vi "Globali.vi"() -> ()   [LabVIEW 2022 SP3]
panel:
  out "Fase Prot35":bool
  out "Fase Scarico":bool
  out "I.A. 4":bool
  out "I.A. 3":bool
  out "I.A. 2":bool
  out "I.A. 1":bool
  in  "copia dati report":string[](array[string])
  in  "Dati_report":string[](array[string])
  in  "Ore manut.":i16
  in  "Militare":bool
  out "t. tot.":i32 format="%<%H:%M:%S>t"
  out "t. Step":i32 format="%<%H:%M:%S>t"
  out "PASS MAN.":string
  in  "Tipo":i16
  out "F.1_NOK_PERDITE_OLIO":bool
  out "F.1_OK_PERDITE_OLIO":bool
  out "PR.1_OK_RUMORE":bool
  out "prod/ric/rev":string
  out "PASS OPER.":string
  out "PASS AMM.":string
  out "m_tipo":u32
  out "m_start":bool
  out "m_tempo":bool
  out "m_numero cicli":bool
  out "m_1 avvio":bool
  out "Scrivi":bool
  in  "Autocontrollo":string
  out "In?":bool
  out "Indicazioni":string
  out "O.F.2-2_OK_LAVAGGIO":bool
  out "O.F.2-1_OK_EROGAZ_PROT35":bool
  out "O.F.3_OK_FINE_CICLO":bool
  out "O.F.1-1_OK_EROGAZ_PROD":bool
  out "I.A.2_OK_FLANGIA_BLOCC":bool
  out "I.A.1_OK_FLANGIA_LIBERA":bool
  out "O.P.3_OK_INSER_ASSE":bool
  out "O.P.2_OK_RISCALDO":bool
  out "O.P.1_OK_EROGAZIONE":bool
  out "Directory modelli report":path=path "D:/Archivio/Iveco/074-07/LabView/Appoggio"
  in  "diagnostica":bool
  out "Testo allarmi":string caption="Collaudo in corso"
  out "Testo fase collaudo":string caption="Collaudo in corso"
  out "Testo segnalazioni":string caption="Collaudo in corso"
  out "Testo messaggi":string caption="Collaudo in corso"
  in  "Tab Control":enum32{"SCRITTURA", "LETTURA"}(tab)=enum."LETTURA"
  in  "226. 0":sgl min=0 format="%.2f"
  in  "230. 0":sgl min=0 format="%.2f"
  in  "Calibrazione torsiometro":sgl min=0 format="%.2f"
  in  "VERNICIATO":bool
  in  "OK_MANUTENZIONE":bool
  in  "CONTINUA PROVA":bool
  in  "SOSPENDI PROVA":bool
  in  "ANNULLA PROVA":bool
  in  "2. 5":bool
  in  "0. 0":bool
  in  "0. 1":bool
  in  "0. 2":bool
  in  "0. 3":bool
  in  "0. 4":bool
  in  "0. 5":bool
  in  "0. 6":bool
  in  "0. 7":bool
  in  "1. 0":bool
  in  "1. 1":bool
  in  "1. 2":bool
  in  "1. 3":bool
  in  "1. 4":bool
  in  "1. 5":bool
  in  "1. 6":bool
  in  "1. 7":bool
  in  "2. 0":bool
  in  "2. 1":bool
  in  "2. 2":bool
  in  "2. 3":bool
  in  "2. 4":bool
  in  "4. 0":i16(ring) items=["PRODOTTO", "RP3000", "AAT 2", "AAT 1 3 4"]
  in  "6. 0":i16(ring) items=["TIPO", "PRODUZIONE", "RICAMBIO"]
  in  "8. 0":i16 min=0
  in  "12. 0":sgl min=0 format="%.2f"
  in  "16. 0":i16 min=0
  in  "22. 0":sgl min=0 format="%.2f"
  in  "26. 0":sgl min=0 format="%.2f"
  in  "32. 0":sgl min=0 format="%.2f"
  in  "36. 0":sgl min=0 format="%.2f"
  in  "44. 0":i16 min=0
  in  "50. 0":i16 min=0
  in  "56. 0":i16 min=0
  in  "62. 0":i16 min=0
  in  "68. 0":i16 min=0
  in  "72. 0":sgl min=0 format="%.2f"
  in  "76. 0":sgl min=0 format="%.2f"
  in  "80. 0":sgl min=0 format="%.2f"
  in  "84. 0":i16 min=0
  in  "88. 0":sgl min=0 format="%.2f"
  in  "92. 0":sgl min=0 format="%.2f"
  in  "96. 0":sgl min=0 format="%.2f"
  in  "100. 0":i16 min=0
  in  "104. 0":sgl min=0 format="%.2f"
  in  "108. 0":sgl min=0 format="%.2f"
  in  "112. 0":sgl min=0 format="%.2f"
  in  "116. 0":i16 min=0
  in  "120. 0":sgl min=0 format="%.2f"
  in  "124. 0":sgl min=0 format="%.2f"
  in  "128. 0":sgl min=0 format="%.2f"
  in  "134. 0":sgl min=0 format="%.2f"
  in  "138. 0":sgl min=0 format="%.2f"
  in  "144. 0":i16 min=0
  in  "148. 0":i16 min=0
  in  "154. 0":i16 min=0
  in  "160. 0":sgl min=0 format="%.2f"
  in  "164. 0":sgl min=0 format="%.2f"
  in  "168. 0":sgl min=0 format="%.2f"
  in  "172. 0":i16 min=0
  in  "176. 0":sgl min=0 format="%.2f"
  in  "180. 0":sgl min=0 format="%.2f"
  in  "184. 0":sgl min=0 format="%.2f"
  in  "190. 0":sgl min=0 format="%.2f"
  in  "194. 0":sgl min=0 format="%.2f"
  in  "200. 0":i16 min=0
  in  "206. 0":i16 min=0
  in  "212. 0":i16 min=0
  in  "20. 0":u16
  in  "30. 0":u16
  in  "40. 0":u16
  in  "42. 0":u16
  in  "48. 0":u16
  in  "54. 0":u16
  in  "60. 0":u16
  in  "66. 0":u16
  in  "132. 0":u16
  in  "142. 0":u16
  in  "152. 0":u16
  in  "158. 0":u16
  in  "188. 0":u16
  in  "198. 0":u16
  in  "204. 0":u16
  in  "210. 0":u16
  in  "216. 0":u16
  in  "218. 0":u16
  out "S_VERNICIATO":bool
  out "CICLO_IN_CORSO":bool
  out "S_SCARTO":bool
  out "Cicli_macchina":u16
  out "V_SOVRAPRESSIONE_DX":sgl format="%.2f"
  out "V_SOVRAPRESSIONE_SX":sgl format="%.2f"
  out "S_CANCELLI_CHIUSI":bool
  out "S_CANCELLI_APERTI":bool
  out "S_CARRO_IN_POSIZ_RP3000":bool
  out "S_FILTRO_INTASATO_PROT35":bool
  out "S_FILTRO_INTASATO_RICIRC":bool
  out "V_PERDITA_PRESSURIZZ_DX":sgl format="%.2f"
  out "V_PERDITA_PRESSURIZZ_SX":sgl format="%.2f"
  out "V_PERDITA_GONFIAGGIO_DX":sgl format="%.2f"
  out "V_PERDITA_GONFIAGGIO_SX":sgl format="%.2f"
  out "V_GONFIAGGIO_STAB":sgl format="%.2f"
  out "I1.0-2 EMERGENZA":bool
  out "S_CANCELLO_DX_APERTO":bool
  out "S_CANCELLO_SX_CHIUSO":bool
  out "S_CANCELLO_DX_CHIUSO":bool
  out "S_AUX_ON":bool=TRUE
  out "S_PRESSOSTATO_ARIA":bool
  out "S_CANCELLO_SX_APERTO":bool
  out "S_CANCELLO_SX_SBLOCCATO":bool
  out "S_CANCELLO_DX_SBLOCCATO":bool
  out "S_TRAZIONE_INSERITA":bool
  out "S_SCARICO_A_LAV":bool
  out "S_SCARICO_A_RIP":bool
  out "S_CARRELLO_10W30":bool
  out "S_CARRELLO_W90":bool
  out "S_CARRELLO_PROT35":bool
  out "S_SCARICO_B_LAV":bool
  out "S_SCARICO_B_RIP":bool
  out "S_CARRO_IN_POSIZ_AAT":bool
  out "S_MOTORE_FERMO":bool
  out "C_APERTURA_CANCELLI":bool
  out "C_START_PROVA":bool
  out "C_RESET":bool
  out "C_CHIUSURA_CANCELLI":bool
  out "C_FASE_SUCCESSIVA":bool
  out "S_ALLARME_INVERTER":bool
  out "S_LIVELLO_MIN_10W30":bool
  out "S_LIVELLO_MIN_W90":bool
  out "S_LIVELLO_MIN_PROT35":bool
  out "S_FILTRO_INTASATO_10W30":bool
  out "S_FILTRO_INTASATO_W90":bool
  out "S_PERDITA_10W30":bool
  out "S_PERDITA_W90":bool
  out "S_PERDITA_PROT35":bool
  out "S_TERMICA_10W30":bool
  out "S_TERMICA_W90":bool
  out "S_TERMICA_PROT35":bool
  out "S_TERMICA_RICIRCOLO":bool
  out "CARICO_ARIA_6_BAR":bool
  out "SCARICO_ARIA_6_BAR":bool
  out "CARICO_PRESSURIZZ":bool
  out "S_PERDITA_VASCA_RACCOLT":bool
  out "SCARICO_PRESSURIZZ":bool
  out "RICIRCOLO_OLIO":bool
  out "ACCENSIONE_AZIONAMENTO":bool
  out "START_MOTORE":bool
  out "POMPA_RICIRCOLO":bool
  out "SCARICO_B":bool
  out "EROGAZIONE_10W30":bool
  out "EROGAZIONE_W90":bool
  out "CHIUSURA_CANCELLI":bool
  out "APERTURA_CANCELLI":bool
  out "SCARICO_A":bool
  out "EROGAZIONE_PROT35":bool
  out "ROTAZIONE_SX":bool
  out "SBLOCCO_CANCELLI":bool
  out "LAMPADA_TRAZIONE_ON":bool
  out "POMPA_10W30":bool
  out "POMPA_W90":bool
  out "POMPA_PROT35":bool
  out "LAMPADA_ROSSA":bool
  out "LAMPADA_GIALLA":bool
  out "LAMPADA_VERDE":bool
  out "CICALINO":bool
  out "S_MAN":bool
  out "S_AUTO":bool
  out "mA_RICIRCOLO_OK":bool
  out "mA_RISCALDAMENTO_OK":bool
  out "mA_PRESS_INSERZ_ASSE_OK":bool
  out "mA_TRAZIONE_INSERITA":bool
  out "mA_TRAZIONE_DISINSERITA":bool
  out "mA_RODAGGIO_OK":bool
  out "mA_COPPIA_1_FUN_OK":bool
  out "mA_RICIRCOLO_1_FUN_OK":bool
  out "mA_COPPIA_2_FUN_OK":bool
  out "mA_RICIRCOLO_2_FUN_OK":bool
  out "mA_COPPIA_3_FUN_OK":bool
  out "S_ALLARME":bool
  out "mA_RICIRCOLO_3_FUN_OK":bool
  out "mA_GONFIAGGIO_OK":bool
  out "mA_PERDITE_DX_OK":bool
  out "mA_PERDITE_SX_OK":bool
  out "mA_COPPIA_4_FUN_OK":bool
  out "mA_RICIRCOLO_4_FUN_OK":bool
  out "mA_COPPIA_5_FUN_OK":bool
  out "mA_RICIRCOLO_5_FUN_OK":bool
  out "mA_PRESS_PRESSURIZZ_OK":bool
  out "mA_PRESSURIZZ_DX_OK":bool
  out "mA_PRESSURIZZ_SX_OK":bool
  out "V_TEMP_AMBIENTE":sgl format="%.2f"
  out "V_TEMP_OLIO_AAT_2":sgl format="%.2f"
  out "V_TEMP_OLIO_AAT_1_3_4":sgl format="%.2f"
  out "V_TEMP_CUSCINETTO_AAT":sgl format="%.2f"
  out "V_TEMP_OLIO_RP3000":sgl format="%.2f"
  out "V_TEMP_OLIO_10W30":sgl format="%.2f"
  out "V_TEMP_OLIO_10W90":sgl format="%.2f"
  out "V_PRESS_ARIA_6_BAR":sgl format="%.2f"
  out "V_PRESSURIZZAZIONE":sgl format="%.2f"
  out "V_PRESS_OLIO_RICIRCOLO":sgl format="%.2f"
  out "V_PORTATA_RICIRCOLO":sgl format="%.2f"
  out "V_COPPIA_ASSE_TRASCINAM":sgl format="%.2f"
  out "V_TEMP_OLIO_ROD":sgl format="%.2f"
  out "V_TEMP_OLIO_1_FUN":sgl format="%.2f"
  out "V_COPPIA_1_FUN":sgl format="%.2f"
  out "V_TEMP_CUSCIN_1_FUN_AAT":sgl format="%.2f"
  out "V_PRES_OLIO_RICIRC_1_FUN":sgl format="%.2f"
  out "V_PORT_RICIRC_1_FUN_AAT2":sgl format="%.2f"
  out "V_TEMP_OLIO_2_FUN":sgl format="%.2f"
  out "V_COPPIA_2_FUN":sgl format="%.2f"
  out "V_TEMP_CUSCIN_2_FUN_AAT":sgl format="%.2f"
  out "V_PRES_OLIO_RICIRC_2_FUN":sgl format="%.2f"
  out "V_PORT_RICIRC_2_FUN_AAT2":sgl format="%.2f"
  out "V_TEMP_OLIO_3_FUN":sgl format="%.2f"
  out "V_COPPIA_3_FUN":sgl format="%.2f"
  out "V_TEMP_CUSCIN_3_FUN_AAT":sgl format="%.2f"
  out "V_PRES_OLIO_RICIRC_3_FUN":sgl format="%.2f"
  out "V_PORT_RICIRC_3_FUN_AAT2":sgl format="%.2f"
  out "V_TEMP_OLIO_4_FUN":sgl format="%.2f"
  out "V_COPPIA_4_FUN":sgl format="%.2f"
  out "V_TEMP_CUSCIN_4_FUN_AAT":sgl format="%.2f"
  out "V_PRES_OLIO_RICIRC_4_FUN":sgl format="%.2f"
  out "V_PORT_RICIRC_4_FUN_AAT2":sgl format="%.2f"
  out "V_TEMP_OLIO_5_FUN":sgl format="%.2f"
  out "V_COPPIA_5_FUN":sgl format="%.2f"
  out "V_TEMP_CUSCIN_5_FUN_AAT":sgl format="%.2f"
  out "V_PRES_OLIO_RICIRC_5_FUN":sgl format="%.2f"
  out "V_PORT_RICIRC_5_FUN_AAT2":sgl format="%.2f"
  out "V_PRESS_PRESSURIZZ":sgl format="%.2f"
  out "Messaggi":u16
  out "Segnalazioni":u16
  out "Allarmi":u16
  out "Fase_collaudo":u16
  out "VI_VEL_MOT":u16
  out "VO_VEL_MOT":u16
  out "VI_COPPIA_MOT":u16
  out "CALIBRAZIONE_TORSIOMETRO":bool
  out "S_CANCELLO_CHIUSURA":bool
  out "S_CANCELLO_APERTURA":bool
  out "S_PAUSA":bool
  in  "PC->PLC":bool[][](array[boolean])
  out "PLC->PC":u16[](array[numeric])
  out "Directory sorgente":path=path "D:/Archivio/Iveco/074-07"
  out "Table":string[][](table)
  out "Prodotto":string
  out "Codice scarto":u16[](array[numeric])
  in  "debug":bool
  out "Part number":string
  out "Istante inizio ciclo":timestamp
  out "Nome File Dati":string
  out "Scarto":bool
  out "Misure":string[](array[string])
  in  "STAMPA ETICHETTA":bool=TRUE
  out "Tipo specifica":string
  in  "Workfile.dat":string="Workfile.dat"
  out "Directory di lavoro":path=path "D:/Archivio/Iveco/074-07/LabView/Appoggio"
  in  "Scrivi logseriale.txt":bool
  out "Versione SW":dbl=1.0 format="%.2f"
  out "OPERATORE":string
  out "MATRICOLA":string="0"
  in  "stop":bool
  in  "Parametri":enum32{"GENERALI", "OPERAZIONE REPORT"}(tab)=enum."OPERAZIONE REPORT"
  in  "NOME PRODOTTO":string
  in  "Contascarti per codice":u16[](array[numeric])
  in  "Numero operazioni":u16
  out "Descrizione operazione":string[](array[string])
  # "0"
  # "1"
  # "2"
  # "3"
  # "4"
  # "5"
  # "6"
  # "7"
  # "8"
  # "9"
  # "10"
  # "11"
  # "12"
  # "13"
  # "14"
  # "15"
  # "Percorsi"
  # "Impostabili dal file testi"
  # "PRESSURIZZAZIONE"
  # "MANUTENZIONI"
  # "OPERAZIONI FINALI"
  # "INSERIMENTO TRAZIONE ASSE"
  # "OPERAZIONI PRELIMINARI"
  # "K_VEL_MOT_MAN"
  # "K_PRESS_RICIRC_MAX"
  # "K_TEMP_OLIO_4_FUN"
  # "K_TEMP_OLIO_RP_RISC"
  # "K_VEL_MOT_1_FUN"
  # "K_COPPIA_4_FUN_MIN"
  # "K_VEL_MOT_RISC"
  # "K_TEMP_OLIO_1_FUN"
  # "K_COPPIA_4_FUN_MAX"
  # "KT_RISCALDO_AAT"
  # "K_COPPIA_1_FUN_MIN"
  # "K_VEL_MOT_5_FUN"
  # "K_PRESS_OLIO_RICIRC_MIN"
  # "K_COPPIA_1_FUN_MAX"
  # "K_TEMP_OLIO_5_FUN"
  # "K_PRESS_OLIO_RICIRC_MAX"
  # "K_VEL_MOT_2_FUN"
  # "K_COPPIA_5_FUN_MIN"
  # "KT_PRESSURIZZ_INSERZIONE"
  # "K_TEMP_OLIO_2_FUN"
  # "K_COPPIA_5_FUN_MAX"
  # "K_PRESS_INSERZ_ASSE_MIN"
  # "K_COPPIA_2_FUN_MIN"
  # "KT_PRESSURIZZAZIONE"
  # "K_PRESS_INSERZ_ASSE_MAX"
  # "K_COPPIA_2_FUN_MAX"
  # "K_PRESSURIZZAZIONE_MIN"
  # "KT_INSERZIONE_1_ASSE"
  # "K_VEL_MOT_3_FUN"
  # "K_PRESSURIZZAZIONE_MAX"
  # "KT_DISINSERZIONE_1_ASSE"
  # "K_TEMP_OLIO_3_FUN"
  # "KT_STABILIZZ_PRESSURIZZ"
  # "K_VEL_MOT_1_ROD"
  # "K_COPPIA_3_FUN_MIN"
  # "K_VEL_PRESSURIZZ_DX"
  # "KT_1_ROD"
  # "K_COPPIA_3_FUN_MAX"
  # "KT_PRESSURIZZ_DX"
  # "K_VEL_MOT_2_ROD"
  # "KT_GONFIAGGIO"
  # "K_VEL_PRESSURIZZ_SX"
  # "KT_2_ROD"
  # "K_PRESS_GONFIAGGIO_MIN"
  # "KT_PRESSURIZZ_SX"
  # "K_VEL_MOT_3_ROD"
  # "K_PRESS_GONFIAGGIO_MAX"
  # "K_VEL_MOT_PROT35"
  # "KT_3_ROD"
  # "KT_STABILIZZ_GONFIAGGIO"
  # "KT_PROT35_SX"
  # "K_VEL_MOT_4_ROD"
  # "K_VEL_MOT_4_FUN_RP_DX"
  # "KT_PROT35_DX"
  # "KT_4_ROD"
  # "K_VEL_MOT_4_FUN"
  # "CALIBRAZ. TORSIOMETRO (V)"
  # "K_VEL_MOT_5_ROD"
  # "KT_4_FUN_RP_DX"
  # "K_PERD_GONFIAGGIO"
  # "K_TEMP_OLIO_ROD"
  # "K_VEL_MOT_4_FUN_RP_SX"
  # "K_PERD_PRESSURIZZ"
  # "K_PRESS_RICIRC_MIN"
  # "KT_4_FUN_RP_SX"
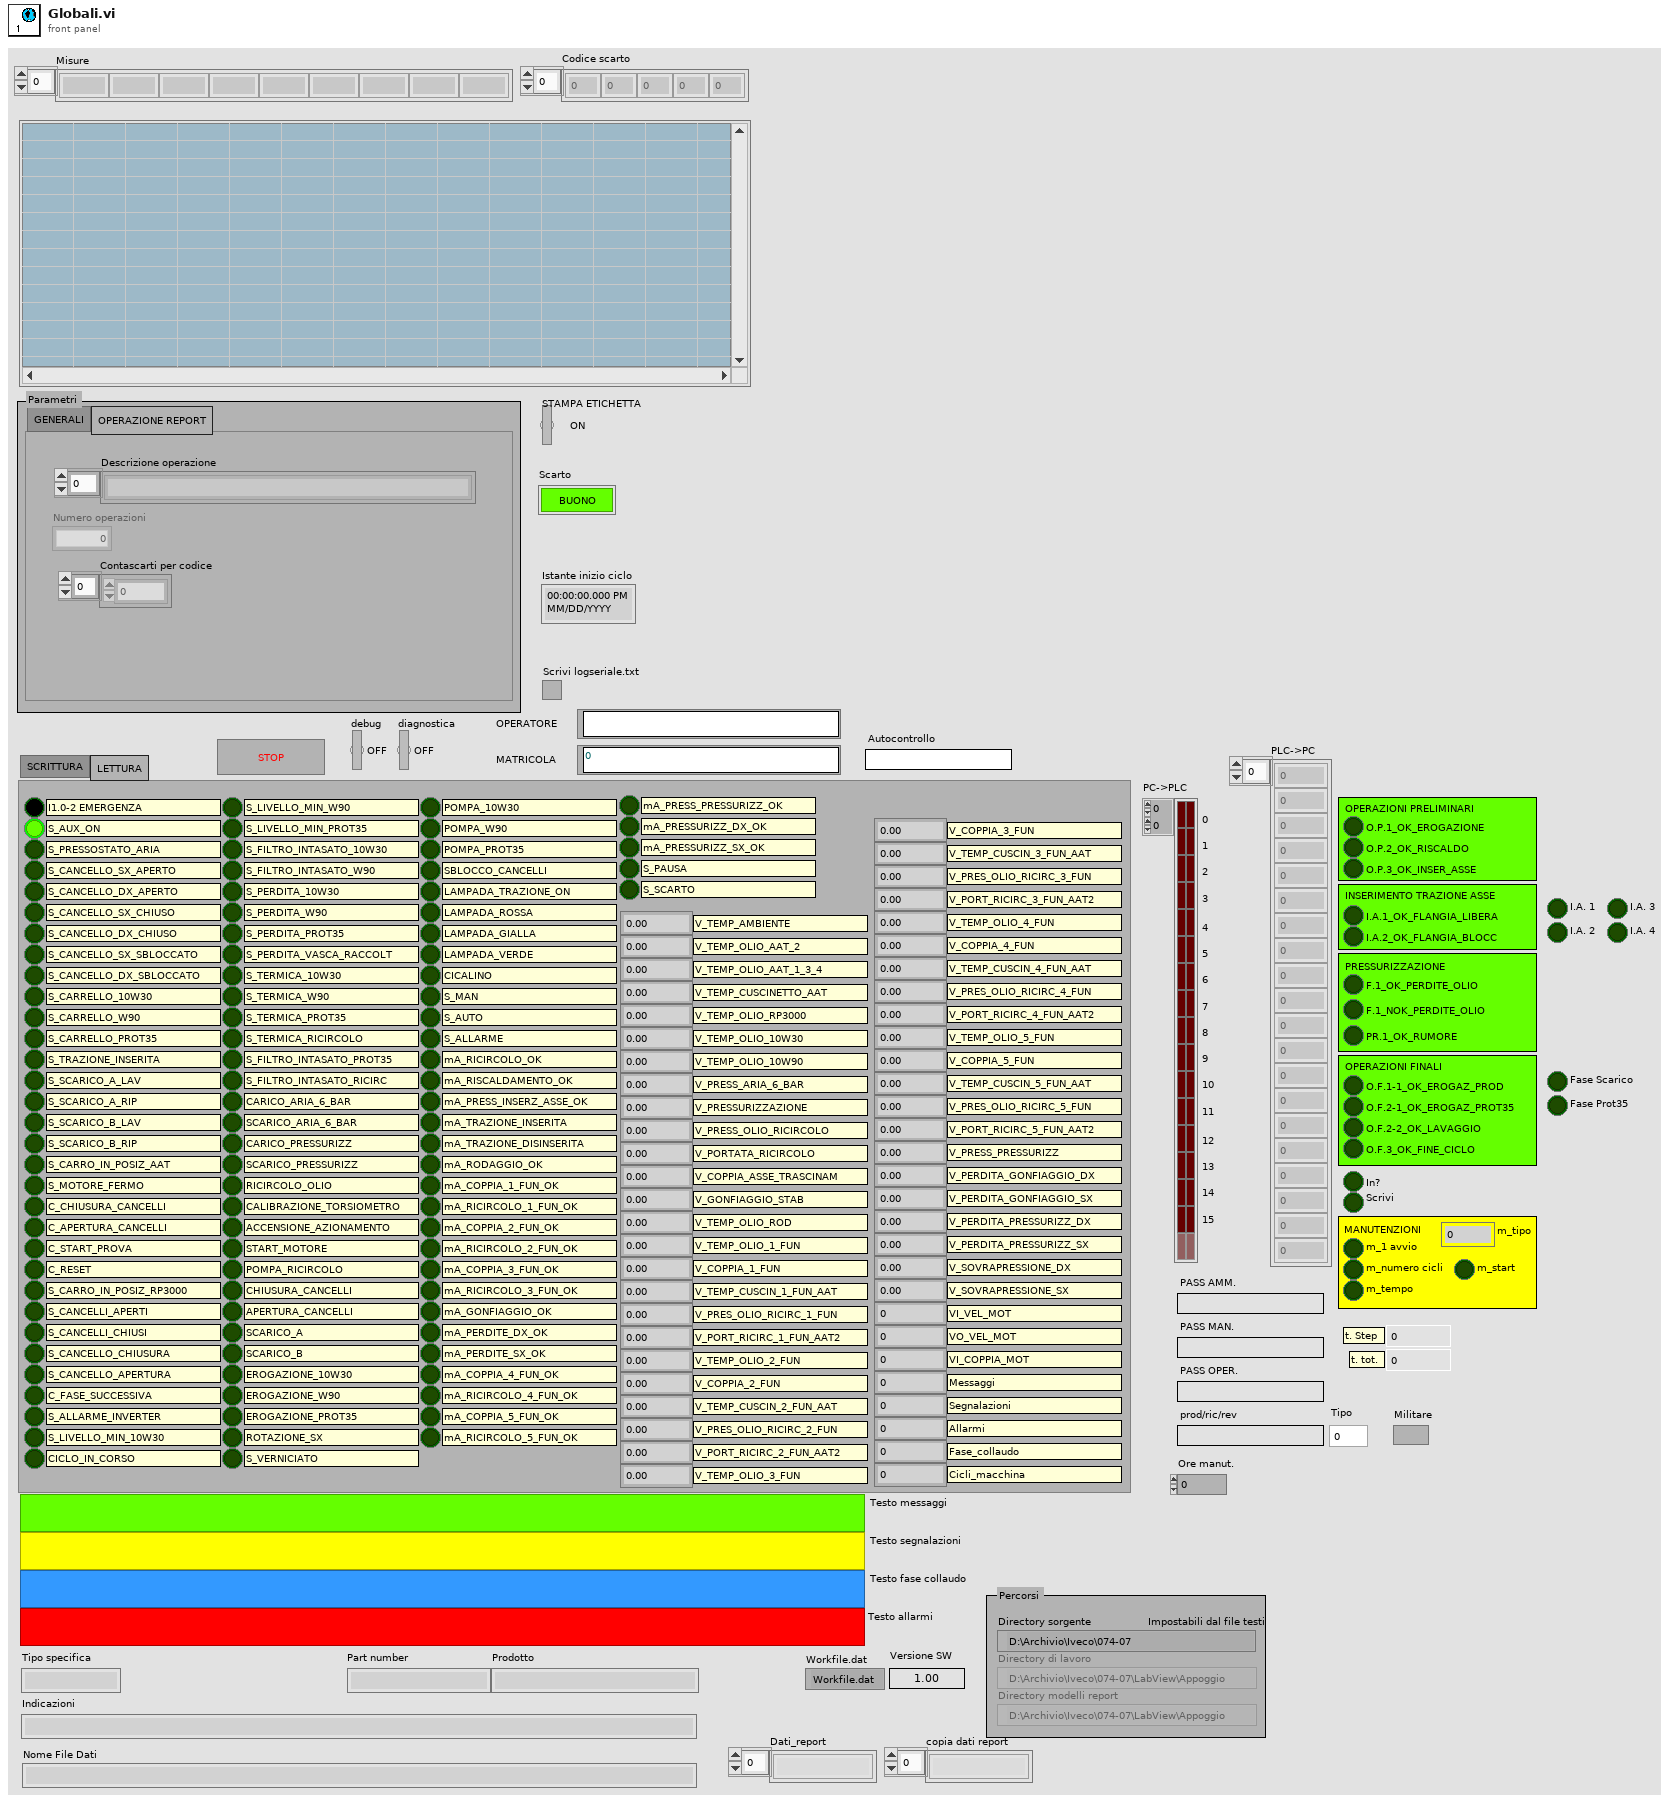
[diagram p1: front panel]
diagram:
